vi "Activate-SM1000-measurement-hardware.vi"(8 "error in (no error)":errorcluster, 11 "SM1000-control in":T1) -> (0 "error out":errorcluster, 1 "Signal":refnum<k21>, 2 "Timing":refnum<k21>, 3 "SM1000-control out":T1, 4 "Batch size":i32)   [LabVIEW 2013, in "MaterialCharacterization.lvlib" / "MC-SM1000.lvclass"]
uses:
  MC-SM1000.lvclass
  Object-reference.ctl
  MC-SM1000.lvclass/MC-SM1000.ctl
  <vilib>/DAQmx/create/channels.llb/DAQmx Create Channel (DI-Digital Input).vi
  <vilib>/DAQmx/create/channels.llb/DAQmx Create Channel (CO-Pulse Generation-Frequency).vi
  <vilib>/DAQmx/configure/timing.llb/DAQmx Timing (Sample Clock).vi
  <vilib>/DAQmx/configure/timing.llb/DAQmx Timing (Implicit).vi
  <resource>/objmgr/daqmx.rc
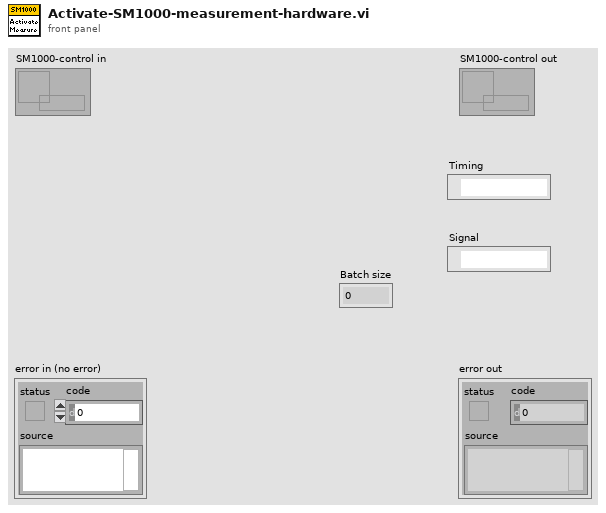
[diagram p1: front panel]
types:
  T1 = typedef "MaterialCharacterization.lvlib/MC-SM1000.lvclass/Object-reference.ctl" = refnum<data-value>
  T2 = typedef "MaterialCharacterization.lvlib/MC-SM1000.lvclass/SM1000-modulation-settings.ctl" = cluster{"Timebase":tag, "Duty cycle":dbl, "Sample rate":dbl, "Batch size":i32, "Timing bypass":tag, "Modulation channel":tag}
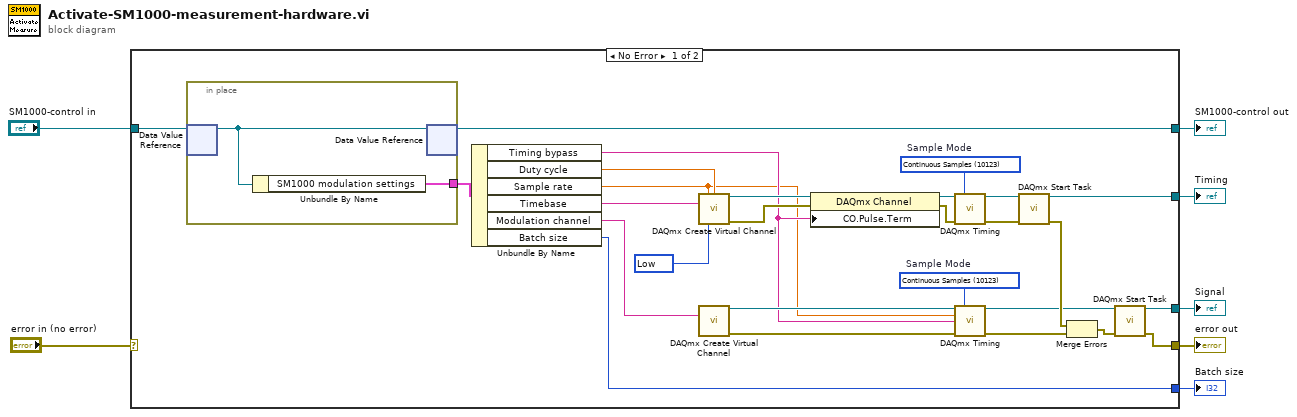
[diagram p0: block diagram]
diagram:
  n1 = case shown="No Error" "error in (no error)" {
    selector: "error in (no error)" -> [_ w38]
    tunnel: [w9 w38] -> w6
    tunnel: [w33 w37] -> w4
    tunnel: "SM1000-control in" -> [w34 w37]
    tunnel: [w11 _] -> w3
    tunnel: [w15 _] -> w2
    tunnel: [w8 _] -> w1
    frame No Error {
      w23 = 10123 items=["Finite Samples"=10178, "Continuous Samples"=10123, "Hardware Timed Single Point"=12522]  # Sample Mode
      w28 = 10123 items=["Finite Samples"=10178, "Continuous Samples"=10123, "Hardware Timed Single Point"=12522]  # Sample Mode
      w29 = 10214 items=["High"=10192, "Low"=10214] ("idle state")
      n2 = in-place {
        in-place-border: [w35] -> w32
        n3 = in-place-dvr #1(w34) -> (w36:refnum<class "MC-SM1000.lvclass">)  [unwired: 1 out]
        n4 = Unbundle By Name(w36) -> ("SM1000 modulation settings"=w35:T2)
        n5 = in-place-dvr #1(w36) -> (w33:T1)  [unwired: 1 out]
      }
      n6 = Unbundle By Name(w32) -> ("Timing bypass"=w21:tag, "Duty cycle"=w31:dbl, "Sample rate"=w20:dbl, "Timebase"=w30:tag, "Modulation channel"=w18:tag, "Batch size"=w8:i32)
      n7 = call-poly <vilib>:"DAQmx Create Virtual Channel.vi"("frequency"=w20, "duty cycle"=w31, "counter"=w30, "idle state"=w29) -> ("task out"=w24:refnum<k21>, "error out"=w27:errorcluster)  [unwired: 10 in]
      n8 = call-poly <vilib>:"DAQmx Create Virtual Channel.vi"("lines"=w18) -> ("task out"=w22:refnum<k21>, "error out"=w19:errorcluster)  [unwired: 13 in]
      n9 = property class="DAQmx Channel"(reference=w24, error in=w27, "CO.Pulse.Term"=w21) -> (reference out=w25:refnum<k21>, error out=w26:errorcluster)
      n10 = call-poly <vilib>:"DAQmx Timing.vi"("task/channels in"=w25, "sample mode"=w28, "error in"=w26) -> ("task out"=w16:refnum<k21>, "error out"=w14:errorcluster)  [unwired: 11 in]
      n11 = call-poly <vilib>:"DAQmx Timing.vi"("task/channels in"=w22, "sample mode"=w23, "rate"=w20, "source"=w21, "error in"=w19) -> ("task out"=w12:refnum<k21>, "error out"=w17:errorcluster)  [unwired: 9 in]
      n12 = call <vilib>:"DAQmx Start Task.vi"("task/channels in"=w16, "error in"=w14) -> ("task out"=w15:refnum<k21>, "error out"=w13:errorcluster)  [unwired: 12 in]
      n13 = Merge Errors(w13, w17) -> (w10:errorcluster)
      n14 = call <vilib>:"DAQmx Start Task.vi"("task/channels in"=w12, "error in"=w10) -> ("task out"=w11:refnum<k21>, "error out"=w9:errorcluster)  [unwired: 12 in]
    }
    frame Error {
    }
  }
  "error out" <- w6
  "SM1000-control out" <- w4
  "Signal" <- w3
  "Timing" <- w2
  "Batch size" <- w1
